vi "fpga_BandPass filter (M Class_50Hz).vi"(0 "input data":fxp<+/-,24,2>, 1 "reset":bool, 5 "Memory In":refnum<k21>="coefROM", 9 "input valid":bool) -> (4 "output data":fxp<+/-,24,3>, 10 "output valid":bool, 14 "ready for input":bool, 15 "error":i32)   [LabVIEW 2013, in "NI_EP_PMU_FPGA.lvlib"]
doc: "----------------------\n\nThis filter is configured as follows:\n\n<b>Filter Configuration</b>\nType: Single Rate\nStructure: FIR Direct Form\n\n<b>Input Data Type</b>\nType: fixed-point <±,24,2> [-2.000000E+0,2.000000E+0]:2.384186E-7\n\n<b>Output Data Type</b>\nType: fixed-point <±,24,3> [-4.000000E+0,4.000000E+0]:4.768372E-7\nRounding mode: Truncate\nOverflow mode: Wrap\n\n<b>Implementation</b>\nNumber of channels: 1\nMaximum input sampling rate per channel @ 40MHz: 32.922kHz\nGain processing: On Host\nMethod: Multiply-Accumulate\nNumber of multiply pipeline stages: 1\nMultiply register in: False\nNumber of adder levels per register: 2\nState memory: Block Memory\nCoefficient memory: Block Memory\n\n<b>Execution Mode</b>\nInside single-cycle Timed Loop\nThroughput: 1215 cycles/sample\n\n<b>Estimated Resources</b>\nNumber of multiply-accumulate units: 1\nMultiply operation: I24.2 x I16.-6 => I40.3"
uses:
  <vilib>/addons/Electrical Power/PMU/NI_EP_PMU_FPGA.lvlib
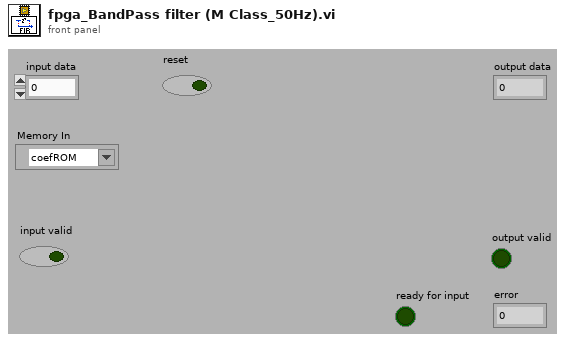
[diagram p1: front panel]
types:
  T1 = cluster{"WREn":bool, "WRAddr":fxp<+,11,11>, "RDAddr":fxp<+,11,11>, "BufWREn":bool, "BufWRAddr":fxp<+,11,11>, "firstRun":bool, "BufFiirstRun":bool}
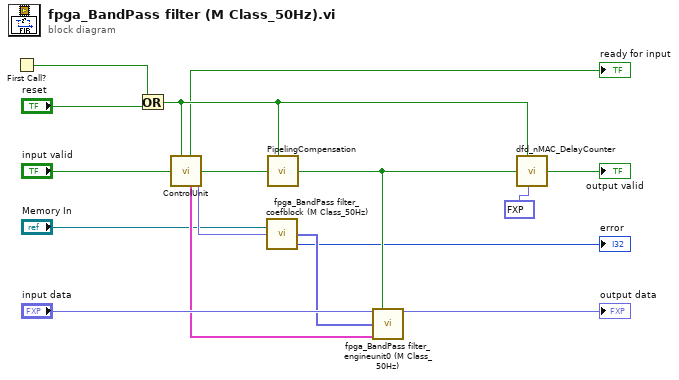
[diagram p0: block diagram]
diagram:
  n1 = First Call?() -> (First Call?: T/F=w13:bool)
  n2 = Or(x=w13, y="reset") -> (x .or. y?=w12:bool)
  n3 = call "ControlUnit"("reset"=w12, "input valid"="input valid") -> ("ready for input"=→"ready for input":bool, "output valid"=w15:bool, "opState"=w8:T1, "coefRDAddr"=w10:fxp<+,11,11>)  [unwired: 4 in]
  n4 = call <vilib>:"fpga_BandPass filter_coefblock (M Class_50Hz).vi"("Memory In"="Memory In", "coefAddr"=w10) -> ("coefficients"=w4:fxp<+/-,18,-4>[], "error"=→"error":i32)  [unwired: 6 in]
  n5 = call "PipelingCompensation"("reset"=w12, "data in"=w15) -> ("data out"=w7:bool)  [unwired: 7 in]
  n6 = call <vilib>:"fpga_BandPass filter_engineunit0 (M Class_50Hz).vi"("input data"="input data", "ACC_Load"=w7, "coefficients"=w4, "opState"=w8) -> ("output data"=→"output data":fxp<+/-,24,3>)  [unwired: 11 in]
  n7 = call "dfd_nMAC_DelayCounter.vi"("reset"=w12, "data in"=w7, "#delay"=fxp<+,11,11> 1215.0 ("#TPPM")) -> ("data out"=→"output valid":bool)  [unwired: 6 in]
